vi "Compute DistanceTo April Tag.vi"(6 "Target Width (in)":dbl=6.5 format="%.1f", 8 "results":T1, 10 "FOV":dbl=68.5, 11 "Image Src":T2) -> (0 "results out":T1, 1 "Off Angle":dbl, 2 "Raw Ball DIstance":dbl, 3 "Image Dst Out":T2, 4 "Distance":dbl)   [LabVIEW 2023]
doc: "Using the camera lens information and the real world size of the target, use trig and ratios to determine the distance to the target. Also returns the location relative to the image center in a (-1 , 1) coordinate system that may be useful for steering the robot."
uses:
  <vilib>/vision/Image Controls.llb/IMAQ Image.ctl
  Vision Support Code/Target Fields.ctl
  <vilib>/ptbypt/NI_PtbyPt.lvlib
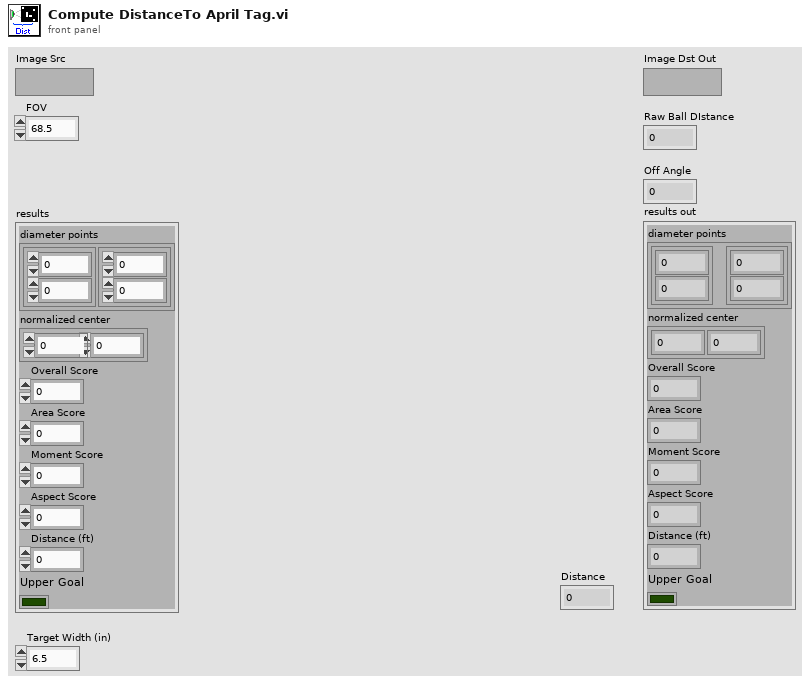
[diagram p1: front panel]
types:
  T1 = typedef "Target Fields.ctl" = cluster{"diameter points":cluster{"first point":cluster{"x":dbl, "y":dbl}, "projected point":cluster{"x":dbl, "y":dbl}}, "normalized center":cluster{"x":dbl, "y":dbl}, "Overall Score":dbl, "Area Score":dbl, "Moment Score":dbl, "Aspect Score":dbl, "Distance (ft)":dbl, "Upper Goal":bool}
  T2 = typedef "IMAQ Image.ctl" = refnum<image>
  T3 = cluster{"first point":cluster{"x":dbl, "y":dbl}, "projected point":cluster{"x":dbl, "y":dbl}}
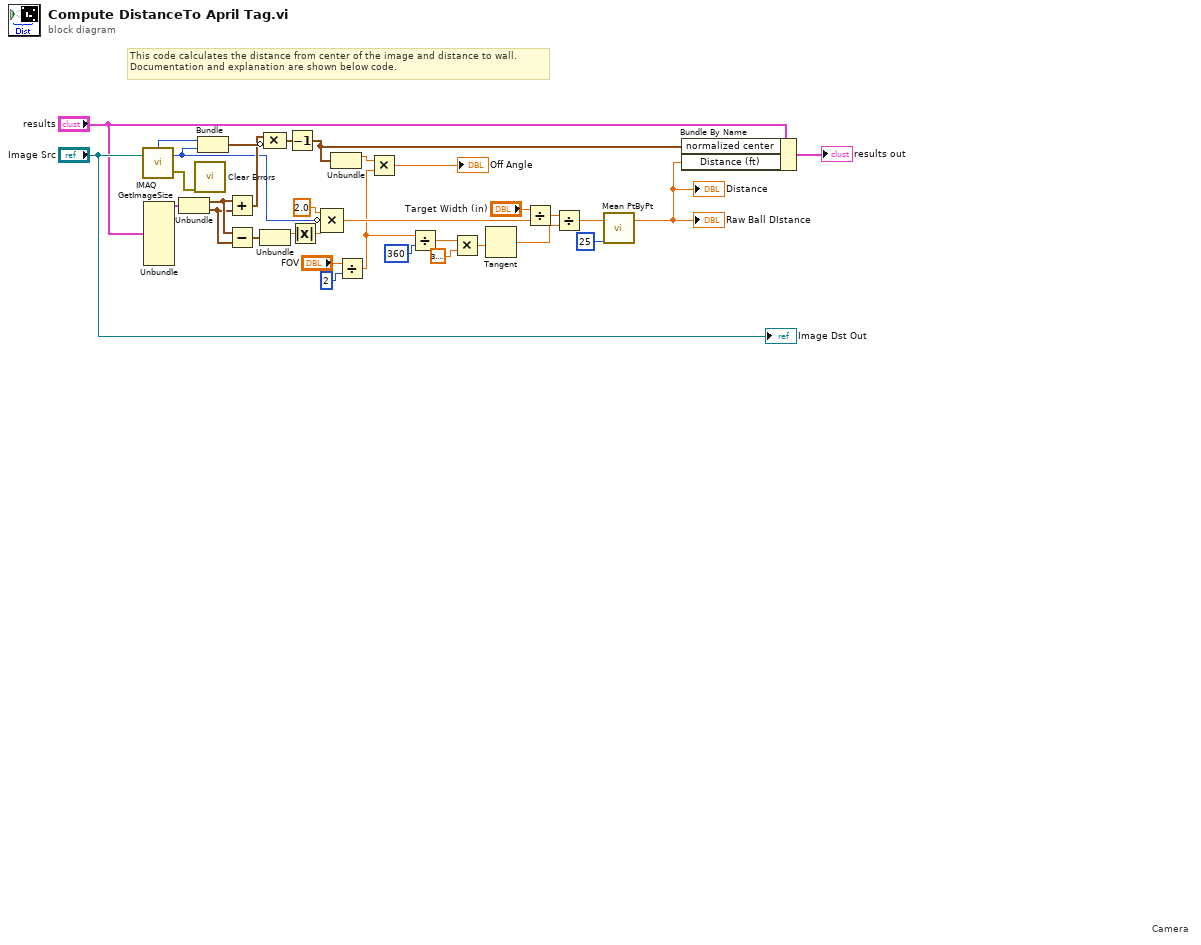
[diagram p0: block diagram]
diagram:
  # "Camera"
  # "This code calculates the distance from center of the image and distance to wall.\nDocumentation and explanation are shown below code."
  n1 = call "IMAQ GetImageSize"("Image"="Image Src") -> ("Y Resolution"=w14:i32, "X Resolution"=w11:i32, "error out"=w25:errorcluster)  [unwired: 3 in]
  n2 = Unbundle("results") -> ("diameter points"=w19:T3)  [unwired: 7 out]
  n3 = Unbundle(w19) -> ("first point"=w17:cluster{"x":dbl, "y":dbl}, "projected point"=w16:cluster{"x":dbl, "y":dbl})
  n4 = call <vilib>:"Clear Errors.vi"("error in (no error)"=w25) -> ()  [unwired: 5 in, 2 out]
  n5 = Bundle("X Resolution"=w11, "Y Resolution"=w14) -> (w18:cluster{"X Resolution":i32, "Y Resolution":i32})  [unwired: 1 in]
  n6 = Add(x=w17, y=w16) -> (x+y=w15:cluster{"x":dbl, "y":dbl})
  n7 = Subtract(x=w17, y=w16) -> (x-y=w1:cluster{"x":dbl, "y":dbl})
  n8 = Unbundle(w1) -> ("x"=w22:dbl)  [unwired: 1 out]
  n9 = Compound Arithmetic op=MULTIPLY(w15, invert w18) -> (w6:cluster{dbl, dbl})
  n10 = Decrement(x=w6) -> (x-1=w12:cluster{dbl, dbl})
  n11 = Absolute Value(x=w22) -> (abs(x)=w23:dbl)
  n12 = Compound Arithmetic op=MULTIPLY(2.0, invert w14, w23) -> (w26:dbl)
  n13 = Unbundle(w12) -> (w10:dbl)  [unwired: 1 out]
  n14 = Divide(x="FOV", y=2) -> (x/y=w5:dbl)
  n15 = Multiply(x=w10, y=w5) -> (x*y=→"Off Angle":dbl)
  n16 = Divide(x=w5, y=360) -> (x/y=w30:dbl)
  n17 = Multiply(x=w30, y=3.141592653589793) -> (x*y=w31:dbl)
  n18 = Tangent(1:w31) -> (0:w28:dbl)
  n19 = Divide(x="Target Width (in)", y=w26) -> (x/y=w9:dbl)
  n20 = Divide(x=w9, y=w28) -> (x/y=w8:dbl)
  n21 = call <vilib>:"Mean PtByPt.vi"("x"=w8, "sample length"=25) -> ("mean"=w4:dbl)  [unwired: 2 in, 1 out]
  "Raw Ball DIstance" <- w4
  "Distance" <- w4
  n22 = Bundle By Name(cluster="results", "normalized center"=w12, "Distance (ft)"=w4) -> (→"results out":T1)
  "Image Dst Out" <- "Image Src"
